vi "Fetch Library Methods Info.vi"(5 "Parser Settings":T9, 8 "Error in":errorcluster caption="Error in (no error)", 11 "Library in":refnum<vi>) -> (0 "Error out":errorcluster, 2 "Methods":T1[](array[typedef]))   [LabVIEW 2023, in "VIDoc Parsing.lvlib" / "Library Documentation.lvclass"]
doc: "Fetches the Library's Method information"
uses:
  Library Documentation.lvclass
  Library Documentation.lvclass/Library Documentation.ctl
  VIDoc Parsing.lvlib
  TypeDefs/VI Type Extended Enum.ctl
  TypeDefs/Class Dispatch Type Enum.ctl
  <vilib>/picture/picture.llb/imagedata.ctl
  <vilib>/Utility/miscctls.llb/LVKeyTypeDef.ctl
  TypeDefs/Controls Info Cluster.ctl
  <vilib>/Utility/miscctls.llb/LVPointTypeDef.ctl
  TypeDefs/Method Spec Cluster.ctl
  Settings/Parser Settings/Draw Option Enum.ctl
  Settings/Parser Settings/Parser Settings.lvclass
  Settings/Parser Settings/Draw Controls Cluster.ctl
  Settings/Parser Settings/Parser Settings Cluster.ctl
  SubVIs/Structure Reporter/Tree Cluster.ctl
  SubVIs/Structure Reporter/Structure Reporter.lvlib
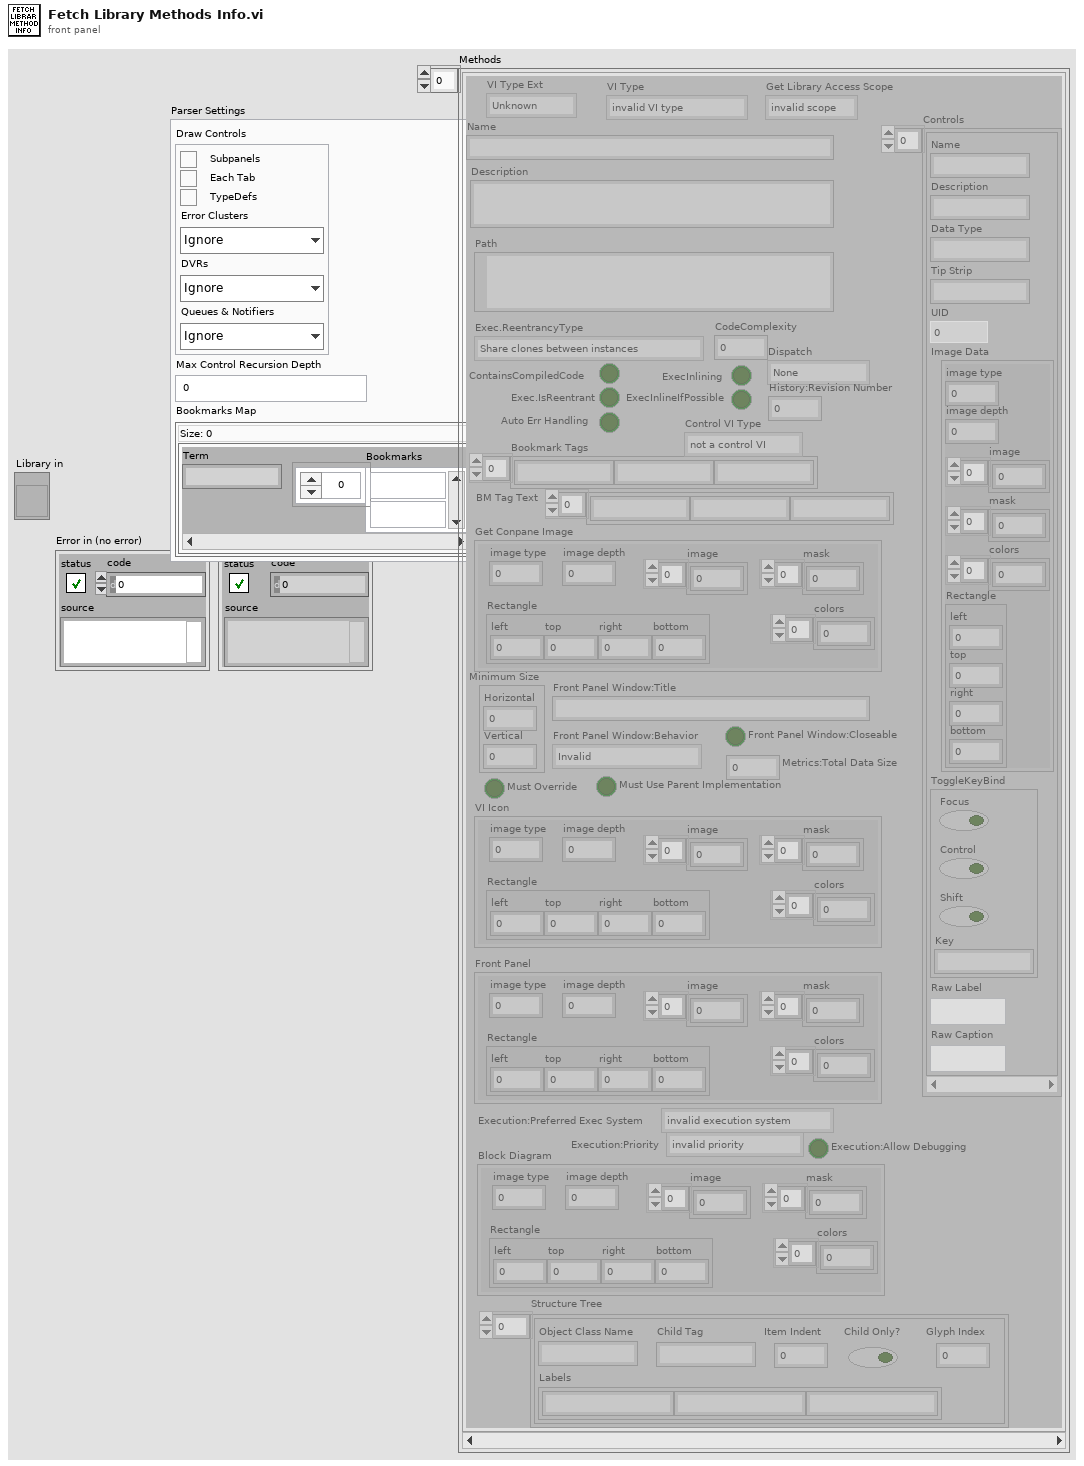
[diagram p1: front panel]
types:
  T1 = typedef "VIDoc Parsing.lvlib/Method Spec Cluster.ctl" = cluster{"VI Type Ext":T2, "Name":string, "Path":path, "Get Conpane Image":T3, "Description":string, "Get Library Access Scope":enum32{"invalid scope", "public", "private", "protected", "community"}, "Dispatch":T4, "ContainsCompiledCode":bool, "Exec.IsReentrant":bool, "Exec.ReentrancyType":enum16{"Share clones between instances", "Preallocate clone for each instance"}, "ExecInlining":bool, "ExecInlineIfPossible":bool, "Auto Err Handling":bool, "CodeComplexity":sgl, "Bookmark Tags":string[], "Control VI Type":enum32{"not a control VI", "control", "typedef", "strict typedef"}, "Controls":T5[], "VI Type":enum32{"invalid VI type", "Standard VI", "Control VI", "Global VI", "Polymorphic VI", "Configuration VI", "SubSystem", "Facade VI", "Method VI", "Statechart Diagram VI"}, "Minimum Size":T7, "Front Panel Window:Title":string, "Front Panel Window:Behavior":enum32{"Invalid", "Default", "Floating", "Floating/Auto-Hide", "Modal"}, "Front Panel Window:Closeable":bool, "Must Override":bool, "Must Use Parent Implementation":bool, "VI Icon":T3, "Front Panel":T3, "History:Revision Number":u32, "Metrics:Total Data Size":u32, "Execution:Allow Debugging":bool, "Execution:Preferred Exec System":enum32{"invalid execution system", "user interface", "standard", "instrument i/o", "data acquisition", "other 1", "other 2", "same as caller"}, "Execution:Priority":enum32{"invalid priority", "background priority", "normal priority", "above normal priority", "high priority", "time critical priority", "subroutine"}, "BM Tag Text":string[], "Block Diagram":T3, "Structure Tree":T8[]}
  T2 = typedef "VIDoc Parsing.lvlib/VI Type Extended Enum.ctl" = enum16{"Unknown", "Class Method", "Class Accessor Get", "Class Accessor Set", "Class Control", "Library Method", "Library Control", "VI", "Control"}
  T3 = typedef "imagedata.ctl" = cluster{"image type":i32, "image depth":i32, "image":u8[], "mask":u8[], "colors":u32[], "Rectangle":cluster{"left":i16, "top":i16, "right":i16, "bottom":i16}}
  T4 = typedef "VIDoc Parsing.lvlib/Class Dispatch Type Enum.ctl" = enum16{"None", "Static", "Dynamic"}
  T5 = typedef "VIDoc Parsing.lvlib/Controls Info Cluster.ctl" = cluster{"Name":string, "Description":string, "Data Type":string, "Tip Strip":string, "UID":i32, "Image Data":T3, "ToggleKeyBind":T6, "Raw Label":string, "Raw Caption":string}
  T6 = typedef "LVKeyTypeDef.ctl" = cluster{"Focus":bool, "Control":bool, "Shift":bool, "Key":string}
  T7 = typedef "LVPointTypeDef.ctl" = cluster{"Horizontal":i16, "Vertical":i16}
  T8 = typedef "VIDoc Parsing.lvlib/Structure Reporter.lvlib/Tree Cluster.ctl" = cluster{"Object Class Name":string, "Labels":string[], "Child Tag":string, "Item Indent":i32, "Child Only?":bool, "Glyph Index":i32}
  T9 = typedef "VIDoc Parsing.lvlib/Parser Settings.lvclass/Parser Settings Cluster.ctl" = cluster{"Draw Controls":T10, "Max Control Recursion Depth":i32, "Bookmarks Map":map{string, string[]}}
  T10 = typedef "VIDoc Parsing.lvlib/Parser Settings.lvclass/Draw Controls Cluster.ctl" = cluster{"Subpanels":bool, "Tabs":bool, "TypeDefs":bool, "Error Clusters":T11, "DVRs":T11, "Queues & Notifiers":T11}
  T11 = typedef "VIDoc Parsing.lvlib/Parser Settings.lvclass/Draw Option Enum.ctl" = enum16{"Ignore", "Draw", "Draw + Contents"}
  T12 = enum32{"invalid VI type", "Standard VI", "Control VI", "Global VI", "Polymorphic VI", "Configuration VI", "SubSystem", "Facade VI", "Method VI", "Statechart Diagram VI"}
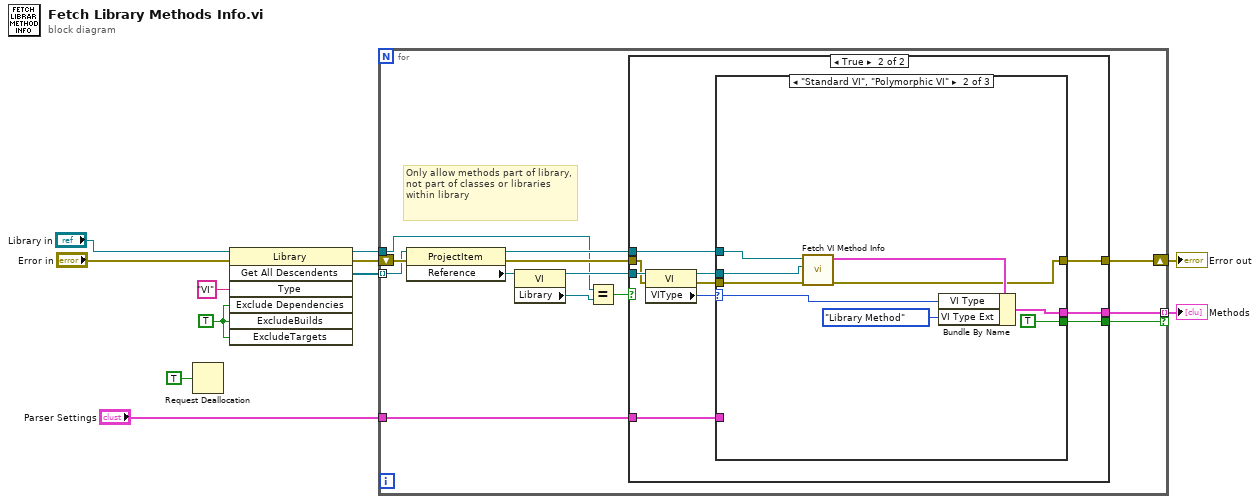
[diagram p0: block diagram]
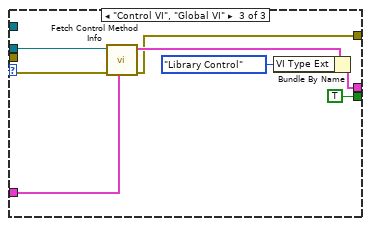
[diagram p4: hidden frame]
diagram:
  w9 = TRUE ("ExcludeDependencies")
  n1 = Request Deallocation(TRUE ("flag")) -> ()
  n2 = invoke class="Library" method="Get All Descendents"(reference="Library in", error in="Error in", "Type"="VI", "Exclude Dependencies"=w9, "ExcludeBuilds"=w9, "ExcludeTargets"=w9) -> (reference out=w8:refnum<vi>, error out=w5:errorcluster, "All Descendents"=w7:refnum<vi>[])  [unwired: 1 in, 4 out]
  n3 = for {
    tunnel: [w24] -> w6 mode=indexing if=w23
    tunnel: w8 -> [w12]
    tunnel: w7 -> [w16] mode=indexing
    shift-right: [w19] -> w4
    shift-left: w5 -> [w21]
    tunnel: "Parser Settings" -> [w18]
    # "Only allow methods part of library, not part of classes or libraries within library"
    n4 = property class="ProjectItem"(reference=w16, error in=w21) -> (reference out=w22:refnum<vi>, error out=w20:errorcluster, "Reference"=w15:refnum<vi>)
    n5 = property class="VI"(reference=w15) -> (reference out=w14:refnum<vi>, "Library"=w13:refnum<vi>)  [unwired: 1 in, 1 out]
    n6 = Equal?(x=w12, y=w13) -> (x = y?=w17:bool)
    n7 = case shown="True" w17 {
      tunnel: [_ w33] -> w24
      tunnel: [_ w32] -> w23
      tunnel: w22 -> [_ w31]
      tunnel: w14 -> [_ w30]
      tunnel: w20 -> [w25 w29]
      tunnel: [w25 w27] -> w19
      tunnel: w18 -> [_ w26]
      frame False {
      }
      frame True {
        n8 = property class="VI"(reference=w30, error in=w29) -> (reference out=w34:refnum<vi>, error out=w28:errorcluster, "VIType"=w35:T12)
        n9 = case shown="\"Standard VI\", \"Polymorphic VI\"" w35 {
          selector: w35 -> [_ w44 _]
          tunnel: w34 -> [_ w37 w51]
          tunnel: w31 -> [_ w42 _]
          tunnel: [_ w43 w47] -> w33
          tunnel: [_ TRUE TRUE] -> w32
          tunnel: w28 -> [w36 w40 w50]
          tunnel: [w36 w39 w49] -> w27
          tunnel: w26 -> [_ _ w48]
          frame Default {
          }
          frame "Standard VI", "Polymorphic VI" {
            n10 = call "Fetch VI Method Info.vi"("Error in"=w40, "VI Reference"=w37, "VI ProjectItem in"=w42) -> ("Error out"=w39:errorcluster, "Method Spec Cluster"=w41:T1)  [unwired: 7 in]
            n11 = Bundle By Name(cluster=w41, "VI Type"=w44, "VI Type Ext"=VI_Type_Extended_Enum."Library Method") -> (w43:T1)
          }
          frame "Control VI", "Global VI" {
            n12 = call "Fetch Control Method Info.vi"("Parser Settings"=w48, "Error in"=w50, "VI in"=w51) -> ("Error out"=w49:errorcluster, "Method Spec Cluster"=w52:T1)  [unwired: 7 in]
            n13 = Bundle By Name(cluster=w52, "VI Type Ext"=VI_Type_Extended_Enum."Library Control") -> (w47:T1)
          }
        }
      }
    }
  }
  "Error out" <- w4
  "Methods" <- w6
